vi "Measure Range.vi"(8 "error in (no error)":errorcluster, 11 "FLS Laser Actor in":refnum<class "FLS Laser Actor.lvclass">) -> (0 "error out":errorcluster, 3 "DLS Laser Actor out":refnum<class "FLS Laser Actor.lvclass">)   [LabVIEW 2018, in "FLS Laser Actor.lvlib" / "FLS Laser Actor.lvclass"]
uses:
  FLS Laser Actor.lvclass
  C:/Program Files (x86)/National Instruments/LabVIEW 2018/vi.lib/ActorFramework/Actor/Actor.lvclass
  FLS Laser Actor.lvclass/FLS Laser Actor.ctl
  <vilib>/ActorFramework/Actor/Actor.lvclass/Actor.ctl
  <vilib>/ActorFramework/Message Enqueuer/Message Enqueuer.lvclass/Message Enqueuer.ctl
  <vilib>/ActorFramework/Message Enqueuer/Init from Existing Queue.vi
  <vilib>/ActorFramework/Message Enqueuer/Enqueue.vi
  <vilib>/ActorFramework/Stop Msg/Stop Msg.lvclass
  C:/Program Files (x86)/National Instruments/LabVIEW 2018/vi.lib/ActorFramework/Message/Message.lvclass
  <vilib>/ActorFramework/Message Priority Queue/Priority Enqueue.vi
  <vilib>/ActorFramework/Message Enqueuer/Message Enqueuer.lvclass
  <vilib>/ActorFramework/Actor/Actor.lvclass
  Range Controller Actor Messages/Send Log Message to Caller Msg/Send Log Message to Caller Msg.lvclass
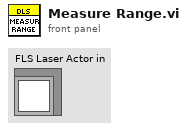
[diagram p1: front panel]
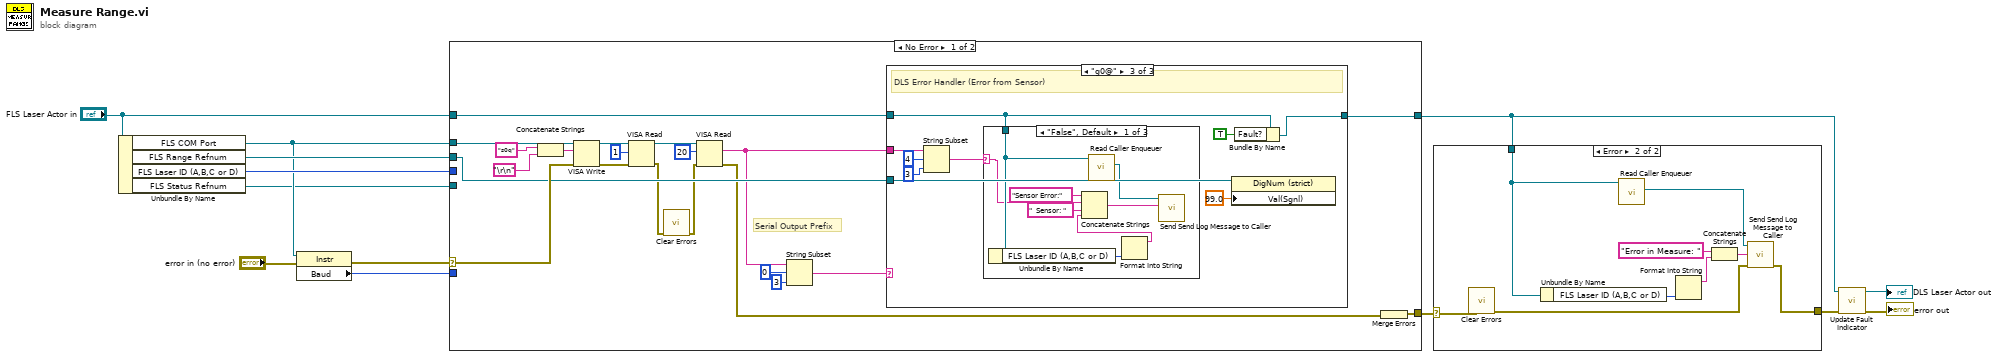
[diagram p0: block diagram]
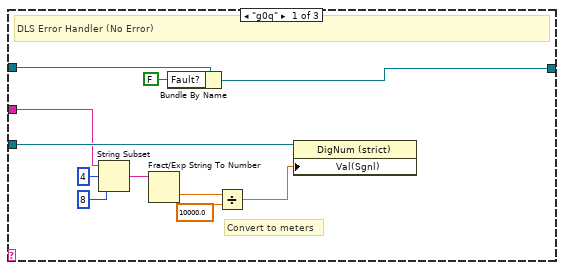
[diagram p3: hidden frame]
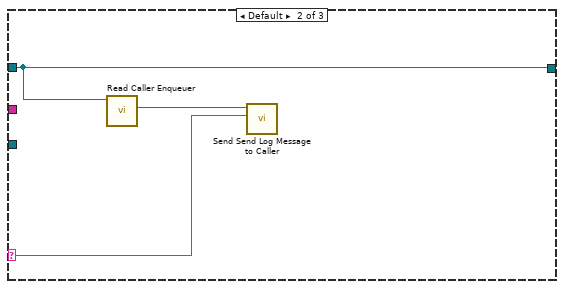
[diagram p4: hidden frame]
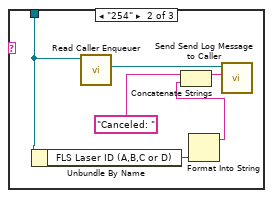
[diagram p5: hidden frame]
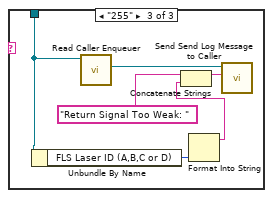
[diagram p6: hidden frame]
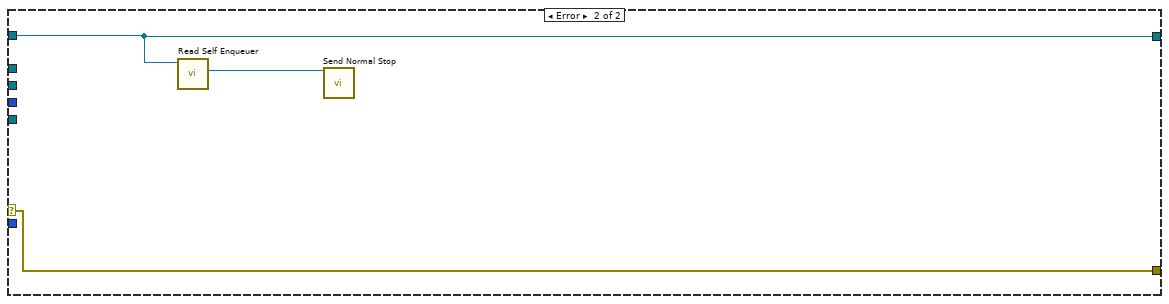
[diagram p7: hidden frame]
diagram:
  n1 = Unbundle By Name("FLS Laser Actor in") -> ("FLS COM Port"=w10:refnum<visa-resource-name>, "FLS Range Refnum"=w13:refnum<vi>, "FLS Laser ID (A,B,C or D)"=w12:enum16{"A", "B", "C", "D"}, "FLS Status Refnum"=w6:refnum<vi>)
  n2 = property class="Instr"(reference=w10, error in="error in (no error)") -> (error out=w8:errorcluster, "Baud"=w7:u32)  [unwired: 1 out]
  n3 = case shown="No Error" w8 {
    selector: w8 -> [w32 w78]
    tunnel: [w26 w80] -> w1
    tunnel: "FLS Laser Actor in" -> [w25 w80]
    tunnel: w10 -> [w33 _]
    tunnel: w13 -> [w31 _]
    tunnel: w12 -> [_ _]
    tunnel: [w30 w78] -> w3
    tunnel: w7 -> [_ _]
    tunnel: w6 -> [_ _]
    frame No Error {
      # "Serial Output Prefix"
      n4 = Concatenate Strings("s0q" ("write buffer"), "\r\n") -> (w28:string)
      n5 = VISA Write(VISA resource name=w33, write buffer=w28, error in (no error)=w32) -> (VISA resource name out=w18:refnum<visa-resource-name>, error out=w16:errorcluster)  [unwired: 1 out]
      n6 = VISA Read(VISA resource name=w18, byte count=u32 1, error in (no error)=w16) -> (VISA resource name out=w17:refnum<visa-resource-name>, error out=w15:errorcluster)  [unwired: 2 out]
      n7 = call <vilib>:"Clear Errors.vi"("error in (no error)"=w15) -> ("error out"=w14:errorcluster)  [unwired: 5 in, 1 out]
      n8 = VISA Read(VISA resource name=w17, byte count=u32 20, error in (no error)=w14) -> (read buffer=w22:string, error out=w20:errorcluster)  [unwired: 2 out]
      n9 = String Subset(string=w22, offset (0)=0, length (rest)=3 ("length (rest)")) -> (substring=w23:string)
      n10 = case shown="\"g0@\"" w23 {
        selector: w23 -> [_ w46 _]
        tunnel: w31 -> [w45 _ w55]
        tunnel: w25 -> [w35 w48 w49]
        tunnel: [w43 w48 w57] -> w26
        tunnel: w22 -> [w38 _ w53]
        frame "g0q" {
          # "Convert to meters"
          # "DLS Error Handler (No Error)"
          n11 = String Subset(string=w38, offset (0)=4, length (rest)=8 ("length (rest)")) -> (substring=w42:string)
          n12 = Fract/Exp String To Number(string=w42) -> (number=w41:dbl)  [unwired: 3 in, 1 out]
          n13 = Bundle By Name(cluster=w35, "Fault?"=FALSE) -> (w43:refnum<class "FLS Laser Actor.lvclass">)
          n14 = Divide(x=w41, y=10000.0) -> (x/y=w36:dbl)
          n15 = property class="DigNum (strict)"(reference=w45, "Val(Sgnl)"=w36) -> ()  [unwired: 1 in, 2 out]
        }
        frame Default {
          n16 = call <vilib>:"Read Caller Enqueuer.vi"("Actor"=w48) -> ("Caller Enqueuer"=w47:refnum<class "Message Enqueuer.lvclass">)  [unwired: 10 in]
          n17 = call "Send Send Log Message to Caller.vi"("Log Message"=w46, "Message Enqueuer in"=w47) -> ()  [unwired: 8 in, 2 out]
        }
        frame "g0@" {
          # "DLS Error Handler (Error from Sensor)"
          n18 = String Subset(string=w53, offset (0)=4 ("length (rest)"), length (rest)=3 ("length (rest)")) -> (substring=w50:string)
          n19 = case shown="\"False\", Default" w50 {
            selector: w50 -> [w60 _ _]
            tunnel: w49 -> [w62 w70 w76]
            frame "False", Default {
              n20 = Unbundle By Name(w62) -> ("FLS Laser ID (A,B,C or D)"=w61:enum16{"A", "B", "C", "D"})
              n21 = call <vilib>:"Read Caller Enqueuer.vi"("Actor"=w62) -> ("Caller Enqueuer"=w65:refnum<class "Message Enqueuer.lvclass">)  [unwired: 10 in]
              n22 = Format Into String(w61) -> (resulting string=w58:string)  [unwired: 3 in, 1 out]
              n23 = Concatenate Strings("Sensor Error:" ("string"), w60, "  Sensor: " ("string"), w58) -> (w64:string)
              n24 = call "Send Send Log Message to Caller.vi"("Log Message"=w64, "Message Enqueuer in"=w65) -> ()  [unwired: 8 in, 2 out]
            }
            frame "254" {
              n25 = Unbundle By Name(w70) -> ("FLS Laser ID (A,B,C or D)"=w69:enum16{"A", "B", "C", "D"})
              n26 = call <vilib>:"Read Caller Enqueuer.vi"("Actor"=w70) -> ("Caller Enqueuer"=w71:refnum<class "Message Enqueuer.lvclass">)  [unwired: 10 in]
              n27 = Format Into String(w69) -> (resulting string=w67:string)  [unwired: 3 in, 1 out]
              n28 = Concatenate Strings("Canceled: " ("Log Message"), w67) -> (w66:string)
              n29 = call "Send Send Log Message to Caller.vi"("Log Message"=w66, "Message Enqueuer in"=w71) -> ()  [unwired: 8 in, 2 out]
            }
            frame "255" {
              n30 = Unbundle By Name(w76) -> ("FLS Laser ID (A,B,C or D)"=w75:enum16{"A", "B", "C", "D"})
              n31 = call <vilib>:"Read Caller Enqueuer.vi"("Actor"=w76) -> ("Caller Enqueuer"=w77:refnum<class "Message Enqueuer.lvclass">)  [unwired: 10 in]
              n32 = Format Into String(w75) -> (resulting string=w73:string)  [unwired: 3 in, 1 out]
              n33 = Concatenate Strings("Return Signal Too Weak: " ("Log Message"), w73) -> (w72:string)
              n34 = call "Send Send Log Message to Caller.vi"("Log Message"=w72, "Message Enqueuer in"=w77) -> ()  [unwired: 8 in, 2 out]
            }
          }
          n35 = property class="DigNum (strict)"(reference=w55, "Val(Sgnl)"=99.0 ("Value (Signaling)")) -> ()  [unwired: 1 in, 2 out]
          n36 = Bundle By Name(cluster=w49, "Fault?"=TRUE) -> (w57:refnum<class "FLS Laser Actor.lvclass">)
        }
      }
      n37 = Merge Errors(w20) -> (w30:errorcluster)
    }
    frame Error {
      n38 = call <vilib>:"Read Self Enqueuer.vi"("Actor"=w80) -> ("Self Enqueuer"=w79:refnum<class "Message Enqueuer.lvclass">)  [unwired: 10 in]
      n39 = call <vilib>:"Send Normal Stop.vi"("Message Enqueuer"=w79) -> ()  [unwired: 10 in, 1 out]
    }
  }
  n40 = case shown="Error" w3 {
    selector: w3 -> [w81 w89]
    tunnel: w1 -> [_ w83]
    tunnel: [w81 w87] -> w2
    frame No Error {
    }
    frame Error {
      n41 = call <vilib>:"Clear Errors.vi"("error in (no error)"=w89) -> ("error out"=w88:errorcluster)  [unwired: 5 in, 1 out]
      n42 = Unbundle By Name(w83) -> ("FLS Laser ID (A,B,C or D)"=w82:enum16{"A", "B", "C", "D"})
      n43 = call <vilib>:"Read Caller Enqueuer.vi"("Actor"=w83) -> ("Caller Enqueuer"=w90:refnum<class "Message Enqueuer.lvclass">)  [unwired: 10 in]
      n44 = Format Into String(w82) -> (resulting string=w84:string)  [unwired: 3 in, 1 out]
      n45 = Concatenate Strings("Error in Measure: " ("string"), w84) -> (w86:string)
      n46 = call "Send Send Log Message to Caller.vi"("error in (no error)"=w88, "Log Message"=w86, "Message Enqueuer in"=w90) -> ("error out"=w87:errorcluster)  [unwired: 7 in, 1 out]
    }
  }
  n47 = call "Update Fault Indicator.vi"("error in (no error)"=w2, "DLS Laser Actor in"=w1) -> ("error out"=→"error out":errorcluster, "DLS Laser Actor out"=→"DLS Laser Actor out":refnum<class "FLS Laser Actor.lvclass">)  [unwired: 8 in]
